vi "题目6.vi"() -> ()   [LabVIEW 2017]
panel:
  out "平均数":dbl
  out "最小值":dbl
  out "最大值":dbl
  out "波形图":dbl[][](graph)
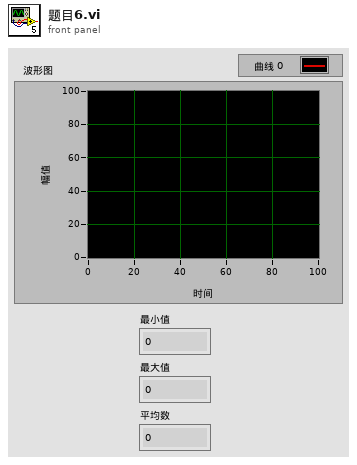
[diagram p1: front panel]
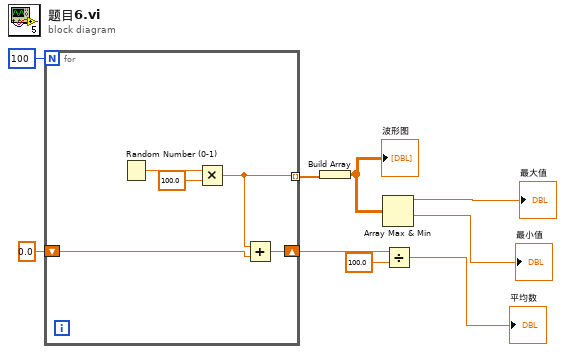
[diagram p0: block diagram]
diagram:
  n1 = for {
    N: 100 -> [_]
    tunnel: [w12] -> w6 mode=indexing
    shift-right: [w11] -> w3
    shift-left: 0.0 -> [w10]
    n2 = Random Number (0-1)() -> (number: 0 to 1=w14:dbl)
    n3 = Multiply(x=w14, y=100.0) -> (x*y=w12:dbl)
    n4 = Add(x=w12, y=w10) -> (x+y=w11:dbl)
  }
  n5 = Build Array(w6) -> (w5:dbl[][])
  "波形图" <- w5
  n6 = Array Max & Min(array=w5) -> (max value=→"最大值":dbl, min value=→"最小值":dbl)  [unwired: 2 out]
  n7 = Divide(x=w3, y=100.0) -> (x/y=→"平均数":dbl)
